vi "Write Typedef Path.vi"(8 "error in (no error)":errorcluster, 10 "Typedef Path":path, 11 "Simple Struct Writer in":refnum<class "Simple Struct Writer.lvclass">) -> (0 "error out":errorcluster, 3 "Simple Struct Writer out":refnum<class "Simple Struct Writer.lvclass">)   [LabVIEW 2013, in "Simple Struct Writer.lvclass"]
doc: "Copyright (c) 2016 Sze Howe Koh\n\nThis Source Code Form is subject to the terms of the Mozilla Public License, v. 2.0. If a copy of the MPL was not distributed with this file, You can obtain one at http://mozilla.org/MPL/2.0/."
uses:
  Simple Struct Writer.lvclass
  Simple Struct Writer.lvclass/Simple Struct Writer.ctl
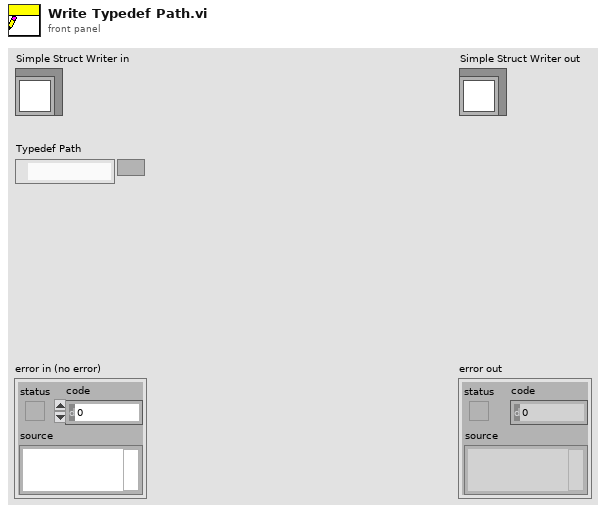
[diagram p1: front panel]
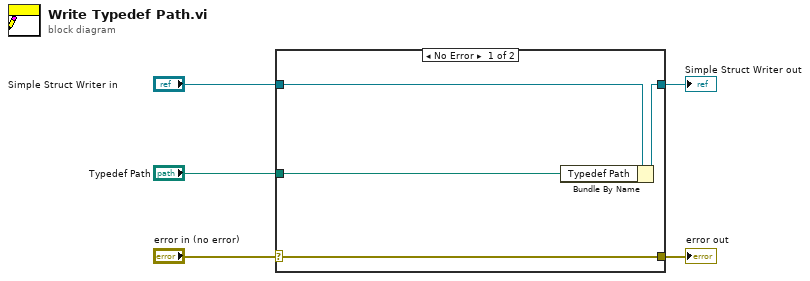
[diagram p0: block diagram]
diagram:
  n1 = case shown="No Error" "error in (no error)" {
    selector: "error in (no error)" -> [w9 w10]
    tunnel: [w9 w10] -> w4
    tunnel: [w7 w11] -> w2
    tunnel: "Simple Struct Writer in" -> [w8 w11]
    tunnel: "Typedef Path" -> [w6 _]
    frame No Error {
      n2 = Bundle By Name(cluster=w8, "Typedef Path"=w6) -> (w7:refnum<class "Simple Struct Writer.lvclass">)
    }
    frame Error {
    }
  }
  "error out" <- w4
  "Simple Struct Writer out" <- w2
